vi "fg_POI max image.vi"(9 "Function":T1, 10 "GreenPOIMax in":T2, 11 "RedPOIMax in":T2) -> (2 "GreenPOIMax out":T2, 3 "RedPOIMax out":T2)   [LabVIEW 2017]
uses:
  <vilib>/vision/Image Controls.llb/IMAQ Image.ctl
  Typedefs/Get-Set-Clear Control.ctl
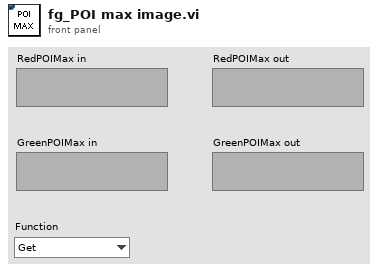
[diagram p1: front panel]
types:
  T1 = typedef "Get-Set-Clear Control.ctl" = enum16{"Get", "Set", "Clear"}
  T2 = typedef "IMAQ Image.ctl" = refnum<image>
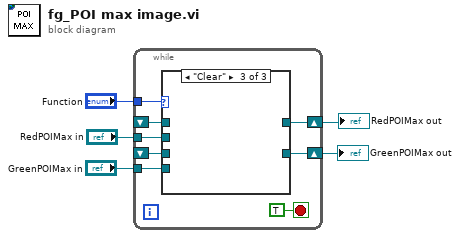
[diagram p0: block diagram]
diagram:
  n1 = while {
    shift-right: [w12] -> w4
    shift-left: _ -> [w8]
    shift-right: [w10] -> w5
    shift-left: _ -> [w7]
    tunnel: "RedPOIMax in" -> [w11]
    tunnel: "GreenPOIMax in" -> [w9]
    tunnel: "Function" -> [w6]
    stop <- TRUE stop-if-true
    n2 = case shown="\"Clear\"" w6 {
      tunnel: [w15 w17 _] -> w12
      tunnel: w11 -> [_ w17 _]
      tunnel: [w14 w16 _] -> w10
      tunnel: w9 -> [_ w16 _]
      tunnel: w8 -> [w15 _ _]
      tunnel: w7 -> [w14 _ _]
      frame "Get", Default {
      }
      frame "Set" {
      }
      frame "Clear" {
      }
    }
  }
  "RedPOIMax out" <- w4
  "GreenPOIMax out" <- w5
